vi "Calcolo Errori.vi"(10 "Misure":T3, 11 "Riferimenti":T2) -> (0 "TVE":waveform(dbl)(graph), 1 "Errore Frequenza":waveform(dbl)(graph), 2 "Errore Fase":waveform(dbl)(graph), 3 "Errore Ampiezza":waveform(dbl)(graph), 4 "Frequenza Misurata":waveform(dbl)[](graph), 5 "Fase Misurata":waveform(dbl)[](graph), 7 "Ampiezza Misurata":waveform(dbl)[](graph))   [LabVIEW 2019]
uses:
  <vilib>/Analysis/coordinate.llb/Wrap Angle (scalar).vi
  <vilib>/Analysis/NI_AAL_Angle.lvlib
panel:
  in  "Tab Control":T1(tab)
  # "QUA INIZIO DA 020 POICHè IL PRIMO VALORE NON AVEVA SENSO POICHè NON POSSO FARE LA DIFFERENZA CON NESSUN VALORE PRECEDENTE E MI DAVA NATURALMENTE ERRORE"
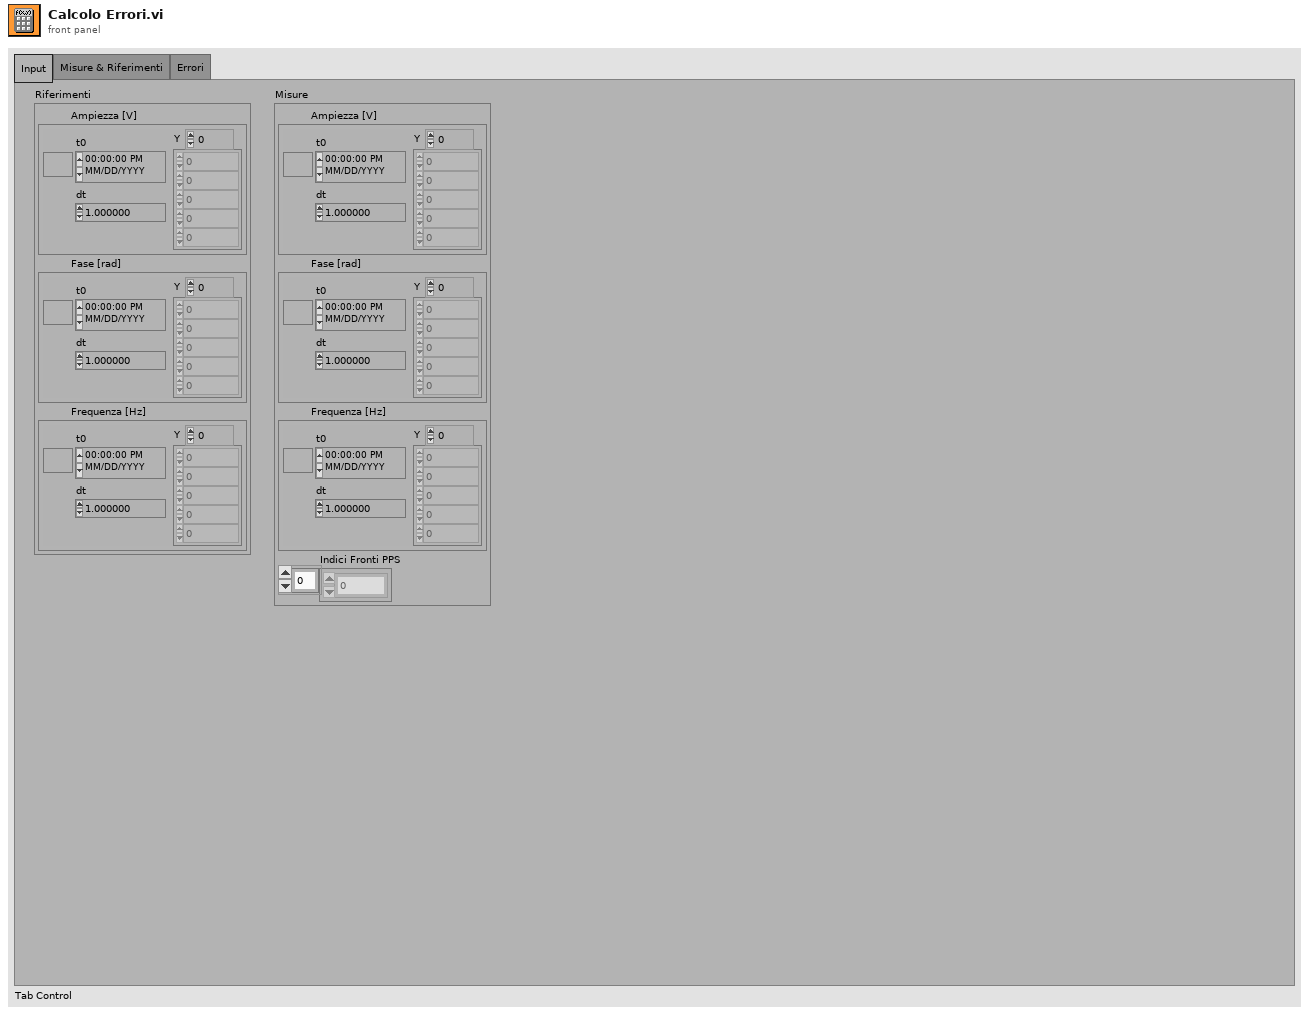
[diagram p1: front panel]
types:
  T1 = enum32{"Input", "Misure & Riferimenti", "Errori"}
  T2 = cluster{"Ampiezza [V]":waveform(dbl), "Fase [rad]":waveform(dbl), "Frequenza [Hz]":waveform(dbl)}
  T3 = cluster{"Ampiezza [V]":waveform(dbl), "Fase [rad]":waveform(dbl), "Frequenza [Hz]":waveform(dbl), "Indici Fronti PPS":i32[]}
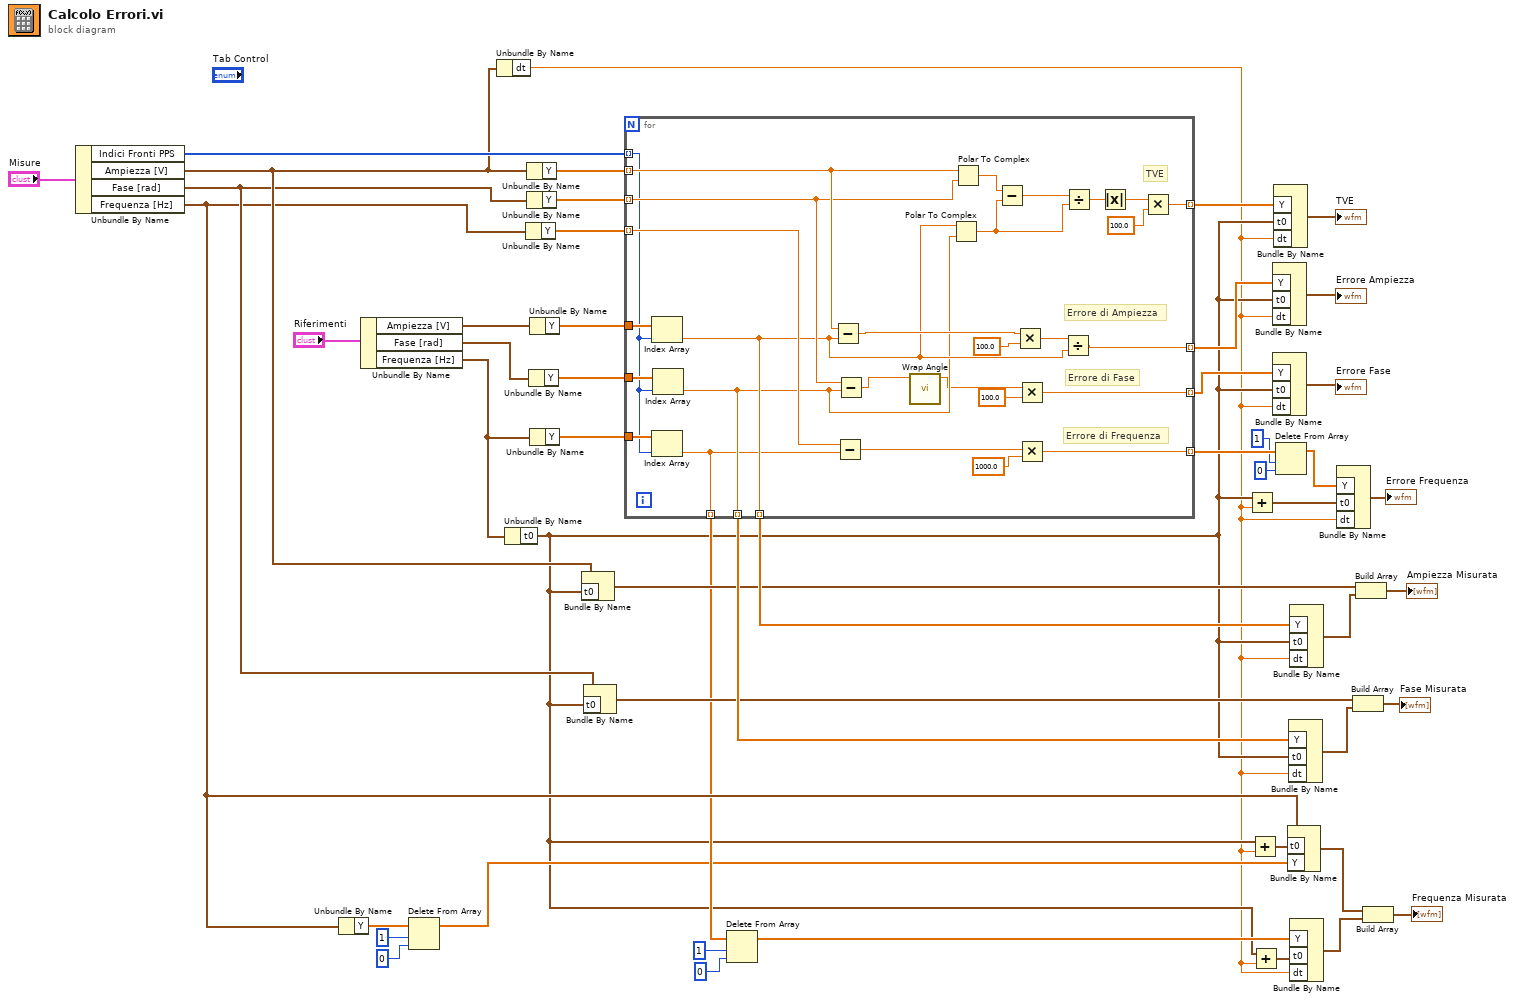
[diagram p0: block diagram]
diagram:
  n1 = Unbundle By Name "Unbundle By Name"("Misure") -> ("Indici Fronti PPS"=w46:i32[], "Ampiezza [V]"=w26:waveform(dbl), "Fase [rad]"=w25:waveform(dbl), "Frequenza [Hz]"=w13:waveform(dbl))
  n2 = Unbundle By Name(w13) -> ("Y"=w12:dbl[])
  n3 = Unbundle By Name "Unbundle By Name"("Riferimenti") -> ("Ampiezza [V]"=w45:waveform(dbl), "Fase [rad]"=w48:waveform(dbl), "Frequenza [Hz]"=w44:waveform(dbl))
  n4 = Delete From Array "Delete From Array"(array=w12, length=1, index=0) -> (array with subset deleted=w5:dbl[])  [unwired: 1 out]
  n5 = Unbundle By Name ("Get Waveform Components")(w26) -> ("dt"=w2:dbl)
  n6 = Unbundle By Name(w44) -> ("t0"=w3:timestamp)
  n7 = Unbundle By Name(w13) -> ("Y"=w47:dbl[])
  n8 = Unbundle By Name(w26) -> ("Y"=w33:dbl[])
  n9 = Unbundle By Name(w25) -> ("Y"=w32:dbl[])
  n10 = Unbundle By Name(w48) -> ("Y"=w34:dbl[])
  n11 = Unbundle By Name(w45) -> ("Y"=w35:dbl[])
  n12 = Unbundle By Name(w44) -> ("Y"=w31:dbl[])
  n13 = Bundle By Name(cluster=w26, "t0"=w3) -> (w19:waveform(dbl))
  n14 = Bundle By Name(cluster=w25, "t0"=w3) -> (w17:waveform(dbl))
  n15 = for {
    tunnel: w35 -> [w78]
    tunnel: w33 -> [w59] mode=indexing
    tunnel: w34 -> [w77]
    tunnel: w31 -> [w76]
    tunnel: w32 -> [w58] mode=indexing
    tunnel: w47 -> [w57] mode=indexing
    tunnel: w46 -> [w53] mode=indexing
    tunnel: [w70] -> w43 mode=indexing
    tunnel: [w60] -> w42 mode=indexing
    tunnel: [w65] -> w41 mode=indexing
    tunnel: [w63] -> w24 mode=indexing
    tunnel: [w56] -> w29 mode=indexing
    tunnel: [w55] -> w30 mode=indexing
    tunnel: [w54] -> w9 mode=indexing
    # "TVE"
    # "Errore di Frequenza"
    # "Errore di Fase"
    # "Errore di Ampiezza"
    n16 = Index Array "Index Array"(array=w78, index=w53) -> (element=w56:dbl)
    n17 = Index Array "Index Array"(array=w76, index=w53) -> (element=w54:dbl)
    n18 = Index Array "Index Array"(array=w77, index=w53) -> (element=w55:dbl)
    n19 = Subtract(x=w59, y=w56) -> (x-y=w68:dbl)
    n20 = Subtract(x=w57, y=w54) -> (x-y=w64:dbl)
    n21 = Subtract(x=w58, y=w55) -> (x-y=w52:dbl)
    n22 = call-poly <vilib>:"Wrap Angle.vi"("angle in"=w52) -> ("angle out"=w51:dbl)  [unwired: 9 in, 1 out]
    n23 = Polar To Complex(1:w55, 2:w56) -> (0:w73:cdb)
    n24 = Polar To Complex(1:w58, 2:w59) -> (0:w75:cdb)
    n25 = Subtract(x=w75, y=w73) -> (x-y=w74:cdb)
    n26 = Multiply(x=w68, y=100.0) -> (x*y=w61:dbl)
    n27 = Multiply(x=w51, y=100.0) -> (x*y=w65:dbl)
    n28 = Multiply(x=w64, y=1000.0) -> (x*y=w63:dbl)
    n29 = Divide(x=w61, y=w56) -> (x/y=w60:dbl)
    n30 = Divide(x=w74, y=w73) -> (x/y=w72:cdb)
    n31 = Absolute Value(x=w72) -> (abs(x)=w71:dbl)
    n32 = Multiply(x=w71, y=100.0) -> (x*y=w70:dbl)
  }
  n33 = Delete From Array "Delete From Array"(array=w9, length=1, index=0) -> (array with subset deleted=w4:dbl[])  [unwired: 1 out]
  n34 = Add(x=w3, y=w2) -> (x+y=w36:timestamp)
  n35 = Add(x=w3, y=w2) -> (x+y=w1:timestamp)
  n36 = Add(x=w3, y=w2) -> (x+y=w6:timestamp)
  n37 = Bundle By Name("Y"=w42, "t0"=w3, "dt"=w2) -> (→"Errore Ampiezza":waveform(dbl))  [unwired: 1 in]
  n38 = Bundle By Name("Y"=w41, "t0"=w3, "dt"=w2) -> (→"Errore Fase":waveform(dbl))  [unwired: 1 in]
  n39 = Bundle By Name("Y"=w43, "t0"=w3, "dt"=w2) -> (→"TVE":waveform(dbl))  [unwired: 1 in]
  n40 = Delete From Array "Delete From Array"(array=w24, length=1, index=0) -> (array with subset deleted=w21:dbl[])  [unwired: 1 out]
  n41 = Bundle By Name(cluster=w13, "t0"=w1, "Y"=w5) -> (w16:waveform(dbl))
  n42 = Bundle By Name("Y"=w30, "t0"=w3, "dt"=w2) -> (w18:waveform(dbl))  [unwired: 1 in]
  n43 = Bundle By Name("Y"=w29, "t0"=w3, "dt"=w2) -> (w20:waveform(dbl))  [unwired: 1 in]
  n44 = Bundle By Name("Y"=w4, "t0"=w6, "dt"=w2) -> (w14:waveform(dbl))  [unwired: 1 in]
  n45 = Bundle By Name("Y"=w21, "t0"=w36, "dt"=w2) -> (→"Errore Frequenza":waveform(dbl))  [unwired: 1 in]
  n46 = Build Array(w17, w18) -> (→"Fase Misurata":waveform(dbl)[])
  n47 = Build Array(w19, w20) -> (→"Ampiezza Misurata":waveform(dbl)[])
  n48 = Build Array(w16, w14) -> (→"Frequenza Misurata":waveform(dbl)[])
